vi "emballage affiche le contenu du carton_FLAT.vi"(0 "Tableau \nlots OUT":string[][](array[string]), 3 "error in":errorcluster caption="entrée d'erreur (pas d'erreur)") -> (6 "error out":errorcluster)   [LabVIEW 2020]
doc: "Affiche les pièces du même type que le produit scanné mais qui ont déjà été emballées.\nOn a la possibilité de les visualiser en sélectionnant le n° de commande et le n° du carton."
uses:
  Modules/FS/60_FS_Controles/60_FS_SetGet.ctl
panel:
  out "Nb total cartons \"théorique\"":i32
  in  "Enregistrer liste par carton (docx)":bool
  in  "Enregistrer liste par carton (txt)":bool
  out "refresh":bool
  in  "Remplacer_Valve":bool
  in  "valider":bool
  out "Total de carton dans la commande":i32
  out "Glissière 2":u8(slide)=100 caption="Identification terminé." scale=0.0..100.0
  in  "DATA cmde":T1={"n°article FAS"="12-216E-01-25 F120023 500mA 10ohm", "n° cmde FAS"="R03844/08-01.01.01", "quantité cmde"="4", "ID LIG cmde"="225540", "n° cmde client"="120565              ", "nom client"="Fluid Automat. Systems GmbH", "n° article client"="21088", "indice revision client"="      ", "société de facturation"="FAS Medic SA                            ", "langue a utiliser"="ALL"}
  out "Tab cmde GPAO":string[][](array[string])=[["12-216C-04521", "EQIFIL ", "104mA    230ohm", "03104/08-05.01.01", "3", "221769", "EMAIL VOM 01.04.08  ", "BLATTY AG", "", "      ", "Fluid Automation Systems SA             ", "ALL", "0"], ["12-216C-04521", "EQIFIL ", "104mA    230ohm", "03128/08-01.01.01", "2", "226006", "RETURN FROM VIASYS2 ", "Fluid Automat. Systems GmbH", "", "      ", "Fluid Automation Systems SA             ", "ALL", "1"], ["12-216C-04521", "EQIFIL ", "104mA    230ohm", "03130/08-01.01.01", "1", "226005", "RETURN FROM VIASYS1 ", "Fluid Automat. Systems GmbH", "", "      ", "Fluid Automation Systems SA             ", "ALL", "1"], ["12-216C-04521", "EQIFIL ", "104mA    230ohm", "03365/08-01.01.01", "4", "225536", "SANS PAPIERS GE     ", "Fluid Automat. Systems GmbH", "", "      ", "Fluid Automation Systems SA             ", "ALL", "1"], ["12-216C-04521", "EQIFIL ", "104mA    230ohm", "03570/08-02.01.01", "100", "225052", "SANS PAPIERS        ", "IMI International Sp. z o.o.", "", "      ", "Fluid Automation Systems SA             ", "ANG", "1"], ["12-216C-04521", "EQIFIL ", "104mA    230ohm", "05066/08-01.01.01", "13", "225726", "120830              ", "Fluid Automat. Systems GmbH", "", "      ", "Fluid Automation Systems SA             ", "ALL", "1"], ["12-216C-04521", "EQIFIL ", "104mA    230ohm", "05067/08-01.01.01", "11", "225727", "120831              ", "Fluid Automat. Systems GmbH", "", "      ", "Fluid Automation Systems SA             ", "ALL", "1"]]
  in  "imprimer étiquette":bool
  out "Nbr valve dans carton/commande":string
  in  "n° commande":string="6340/07-02.01.01"
  out "Pièces dans le carton":i32[](listbox)
  in  "Tableau historique":string[][](array[string])=[["MK0228606ARXA2199", "24.02.2006 11:58", "AFA", "5401/04", "1", "200"], ["MK0228606ARXA2177", "24.02.2006 12:00", "AFA", "5401/04", "1", "200"], ["MK0228606ARXA2178", "24.02.2006 12:00", "AFA", "5401/04", "1", "200"], ["MK0228606ARXA2198", "24.02.2006 12:12", "AFA", "5401/04", "1", "200"], ["MK0228606ARXA2197", "24.02.2006 12:12", "AFA", "5401/04", "1", "200"], ["MK0228606ARXA2196", "24.02.2006 12:13", "AFA", "5401/04", "1", "200"], ["MK0228606ARXA2195", "24.02.2006 12:13", "AFA", "5401/04", "1", "200"], ["MK0228606ARXA2176", "24.02.2006 12:13", "AFA", "5401/04", "1", "200"], ["MK0228606ARXA2194", "24.02.2006 12:13", "AFA", "5401/04", "1", "200"], ["MK0228606ARXA2193", "24.02.2006 12:13", "AFA", "5401/04", "1", "200"], ["MK0228606ARXA2175", "24.02.2006 12:14", "AFA", "5401/04", "1", "200"], ["MK0228606ARXA2171", "24.02.2006 12:14", "AFA", "5401/04", "1", "200"], ["MK0228606ARXA2174", "24.02.2006 12:14", "AFA", "5401/04", "1", "200"], ["MK0228606ARXA2173", "24.02.2006 12:14", "AFA", "5401/04", "1", "200"], ["MK0228606ARXA2172", "24.02.2006 12:14", "AFA", "5401/04", "1", "200"], ["MK0228606ARXA2192", "24.02.2006 12:14", "AFA", "5401/04", "1", "200"], ["MK0228606ARXA2191", "24.02.2006 12:14", "AFA", "5401/04", "1", "200"], ["MK0228606ARXA2190", "24.02.2006 12:14", "AFA", "5401/04", "1", "200"], ["MK0228606ARXA2189", "24.02.2006 12:15", "AFA", "5401/04", "1", "200"], ["MK0228606ARXA2188", "24.02.2006 12:15", "AFA", "5401/04", "1", "200"], ["MK0228606ARXB4259", "09.03.2006 17:40", "AYU", "5401/04-03.03", "5", "300"], ["MK0228606ARXB4258", "09.03.2006 17:40", "AYU", "5401/04-03.03", "5", "300"], ["MK0228606ARXB4257", "09.03.2006 17:40", "AYU", "5401/04-03.03", "5", "300"], ["MK0228606ARXB4256", "09.03.2006 17:39", "AYU", "5401/04-03.03", "5", "300"], ["MK0228606ARXB4255", "09.03.2006 17:39", "AYU", "5401/04-03.03", "5", "300"], ["MK0228606ARXB4254", "09.03.2006 17:39", "AYU", "5401/04-03.03", "5", "300"], ["MK0228606ARXB4253", "09.03.2006 17:39", "AYU", "5401/04-03.03", "5", "300"], ["MK0228606ARXB4252", "09.03.2006 17:39", "AYU", "5401/04-03.03", "5", "300"], ["MK0228606ARXB4251", "09.03.2006 17:39", "AYU", "5401/04-03.03", "5", "300"], ["MK0228606ARXB4250", "09.03.2006 17:39", "AYU", "5401/04-03.03", "5", "300"], ["MK0228606ARXB4249", "09.03.2006 17:39", "AYU", "5401/04-03.03", "5", "300"], ["MK0228606ARXB4248", "09.03.2006 17:39", "AYU", "5401/04-03.03", "5", "300"], ["MK0228606ARXB4247", "09.03.2006 17:39", "AYU", "5401/04-03.03", "5", "300"], ["MK0228606ARXB4246", "09.03.2006 17:39", "AYU", "5401/04-03.03", "5", "300"], ["MK0228606ARXB4245", "09.03.2006 17:38", "AYU", "5401/04-03.03", "5", "300"], ["MK0228606ARXB4244", "09.03.2006 17:38", "AYU", "5401/04-03.03", "5", "300"], ["MK0228606ARXB4243", "09.03.2006 17:38", "AYU", "5401/04-03.03", "5", "300"], ["MK0228606ARXB4242", "09.03.2006 17:38", "AYU", "5401/04-03.03", "5", "300"], ["MK0228606ARXB4241", "09.03.2006 17:38", "AYU", "5401/04-03.03", "5", "300"], ["MK0228606ARXB4240", "09.03.2006 17:38", "AYU", "5401/04-03.03", "5", "300"], ["MK0228606ARXB4239", "09.03.2006 17:33", "AYU", "5401/04-03.03", "4", "300"], ["MK0228606ARXB4238", "09.03.2006 17:32", "AYU", "5401/04-03.03", "4", "300"], ["MK0228606ARXB4237", "09.03.2006 17:32", "AYU", "5401/04-03.03", "4", "300"], ["MK0228606ARXB4236", "09.03.2006 17:32", "AYU", "5401/04-03.03", "4", "300"], ["MK0228606ARXB4235", "09.03.2006 17:32", "AYU", "5401/04-03.03", "4", "300"], ["MK0228606ARXB4234", "09.03.2006 17:32", "AYU", "5401/04-03.03", "4", "300"], ["MK0228606ARXB4233", "09.03.2006 17:32", "AYU", "5401/04-03.03", "4", "300"], ["MK0228606ARXB4232", "09.03.2006 17:32", "AYU", "5401/04-03.03", "4", "300"], ["MK0228606ARXB4231", "09.03.2006 17:31", "AYU", "5401/04-03.03", "4", "300"], ["MK0228606ARXB4230", "09.03.2006 17:31", "AYU", "5401/04-03.03", "4", "300"], ["MK0228606ARXB4229", "09.03.2006 17:31", "AYU", "5401/04-03.03", "4", "300"], ["MK0228606ARXB4228", "09.03.2006 17:31", "AYU", "5401/04-03.03", "4", "300"], ["MK0228606ARXB4227", "09.03.2006 17:31", "AYU", "5401/04-03.03", "4", "300"], ["MK0228606ARXB4226", "09.03.2006 17:31", "AYU", "5401/04-03.03", "4", "300"], ["MK0228606ARXB4225", "09.03.2006 17:30", "AYU", "5401/04-03.03", "4", "300"], ["MK0228606ARXB4224", "09.03.2006 17:30", "AYU", "5401/04-03.03", "4", "300"], ["MK0228606ARXB4223", "09.03.2006 17:30", "AYU", "5401/04-03.03", "4", "300"], ["MK0228606ARXB4222", "09.03.2006 17:30", "AYU", "5401/04-03.03", "4", "300"], ["MK0228606ARXB4221", "09.03.2006 17:30", "AYU", "5401/04-03.03", "4", "300"], ["MK0228606ARXB4220", "09.03.2006 17:30", "AYU", "5401/04-03.03", "4", "300"], ["MK0228606ARXB4219", "09.03.2006 17:24", "AYU", "5401/04-03.03", "3", "300"], ["MK0228606ARXB4218", "09.03.2006 17:23", "AYU", "5401/04-03.03", "3", "300"], ["MK0228606ARXB4217", "09.03.2006 17:23", "AYU", "5401/04-03.03", "3", "300"], ["MK0228606ARXB4216", "09.03.2006 17:23", "AYU", "5401/04-03.03", "3", "300"], ["MK0228606ARXB4215", "09.03.2006 17:23", "AYU", "5401/04-03.03", "3", "300"], ["MK0228606ARXB4214", "09.03.2006 17:23", "AYU", "5401/04-03.03", "3", "300"], ["MK0228606ARXB4213", "09.03.2006 17:23", "AYU", "5401/04-03.03", "3", "300"], ["MK0228606ARXB4212", "09.03.2006 17:22", "AYU", "5401/04-03.03", "3", "300"], ["MK0228606ARXB4211", "09.03.2006 17:21", "AYU", "5401/04-03.03", "3", "300"], ["MK0228606ARXB4210", "09.03.2006 17:21", "AYU", "5401/04-03.03", "3", "300"], ["MK0228606ARXB4209", "09.03.2006 17:21", "AYU", "5401/04-03.03", "3", "300"], ["MK0228606ARXB4208", "09.03.2006 17:20", "AYU", "5401/04-03.03", "3", "300"], ["MK0228606ARXB4207", "09.03.2006 17:20", "AYU", "5401/04-03.03", "3", "300"], ["MK0228606ARXB4206", "09.03.2006 17:20", "AYU", "5401/04-03.03", "3", "300"], ["MK0228606ARXB4205", "09.03.2006 17:20", "AYU", "5401/04-03.03", "3", "300"], ["MK0228606ARXB4204", "09.03.2006 17:20", "AYU", "5401/04-03.03", "3", "300"], ["MK0228606ARXB4203", "09.03.2006 17:20", "AYU", "5401/04-03.03", "3", "300"], ["MK0228606ARXB4202", "09.03.2006 17:19", "AYU", "5401/04-03.03", "3", "300"], ["MK0228606ARXB4201", "09.03.2006 17:19", "AYU", "5401/04-03.03", "3", "300"], ["MK0228606ARXB4200", "09.03.2006 17:18", "AYU", "5401/04-03.03", "3", "300"], ["MK0228606ARXB4199", "09.03.2006 17:12", "AYU", "5401/04-03.03", "2", "300"], ["MK0228606ARXB4198", "09.03.2006 17:11", "AYU", "5401/04-03.03", "2", "300"], ["MK0228606ARXB4197", "09.03.2006 17:11", "AYU", "5401/04-03.03", "2", "300"], ["MK0228606ARXB4196", "09.03.2006 17:11", "AYU", "5401/04-03.03", "2", "300"], ["MK0228606ARXB4195", "09.03.2006 17:11", "AYU", "5401/04-03.03", "2", "300"], ["MK0228606ARXB4194", "09.03.2006 17:11", "AYU", "5401/04-03.03", "2", "300"], ["MK0228606ARXB4193", "09.03.2006 17:11", "AYU", "5401/04-03.03", "2", "300"], ["MK0228606ARXB4192", "09.03.2006 17:10", "AYU", "5401/04-03.03", "2", "300"], ["MK0228606ARXB4191", "09.03.2006 17:10", "AYU", "5401/04-03.03", "2", "300"], ["MK0228606ARXB4190", "09.03.2006 17:10", "AYU", "5401/04-03.03", "2", "300"], ["MK0228606ARXB4189", "09.03.2006 17:10", "AYU", "5401/04-03.03", "2", "300"], ["MK0228606ARXB4188", "09.03.2006 17:10", "AYU", "5401/04-03.03", "2", "300"], ["MK0228606ARXB4187", "09.03.2006 17:10", "AYU", "5401/04-03.03", "2", "300"], ["MK0228606ARXB4186", "09.03.2006 17:10", "AYU", "5401/04-03.03", "2", "300"], ["MK0228606ARXB4185", "09.03.2006 17:10", "AYU", "5401/04-03.03", "2", "300"], ["MK0228606ARXB4184", "09.03.2006 17:09", "AYU", "5401/04-03.03", "2", "300"], ["MK0228606ARXB4183", "09.03.2006 17:09", "AYU", "5401/04-03.03", "2", "300"], ["MK0228606ARXB4182", "09.03.2006 17:09", "AYU", "5401/04-03.03", "2", "300"], ["MK0228606ARXB4181", "09.03.2006 17:08", "AYU", "5401/04-03.03", "2", "300"], ["MK0228606ARXB4180", "09.03.2006 17:08", "AYU", "5401/04-03.03", "2", "300"], ["MK0228606ARXB4179", "09.03.2006 17:01", "AYU", "5401/04-03.03", "1", "300"], ["MK0228606ARXB4178", "09.03.2006 17:01", "AYU", "5401/04-03.03", "1", "300"], ["MK0228606ARXB4177", "09.03.2006 17:01", "AYU", "5401/04-03.03", "1", "300"], ["MK0228606ARXB4176", "09.03.2006 17:01", "AYU", "5401/04-03.03", "1", "300"], ["MK0228606ARXB4175", "09.03.2006 17:00", "AYU", "5401/04-03.03", "1", "300"], ["MK0228606ARXB4174", "09.03.2006 17:00", "AYU", "5401/04-03.03", "1", "300"], ["MK0228606ARXB4173", "09.03.2006 17:00", "AYU", "5401/04-03.03", "1", "300"], ["MK0228606ARXB4172", "09.03.2006 17:00", "AYU", "5401/04-03.03", "1", "300"], ["MK0228606ARXB4171", "09.03.2006 17:00", "AYU", "5401/04-03.03", "1", "300"], ["MK0228606ARXB4170", "09.03.2006 16:57", "AYU", "5401/04-03.03", "1", "300"], ["MK0228606ARXB4169", "09.03.2006 16:57", "AYU", "5401/04-03.03", "1", "300"], ["MK0228606ARXB4168", "09.03.2006 16:56", "AYU", "5401/04-03.03", "1", "300"], ["MK0228606ARXB4167", "09.03.2006 16:56", "AYU", "5401/04-03.03", "1", "300"], ["MK0228606ARXB4166", "09.03.2006 16:56", "AYU", "5401/04-03.03", "1", "300"], ["MK0228606ARXB4165", "09.03.2006 16:55", "AYU", "5401/04-03.03", "1", "300"], ["MK0228606ARXB4164", "09.03.2006 16:55", "AYU", "5401/04-03.03", "1", "300"], ["MK0228606ARXB4163", "09.03.2006 16:55", "AYU", "5401/04-03.03", "1", "300"], ["MK0228606ARXB4162", "09.03.2006 16:54", "AYU", "5401/04-03.03", "1", "300"], ["MK0228606ARXB4161", "09.03.2006 16:54", "AYU", "5401/04-03.03", "1", "300"], ["MK0228606ARXB4160", "09.03.2006 16:52", "AYU", "5401/04-03.03", "1", "300"], ["MK0228606ARXB4158", "10.03.2006 08:35", "AYU", "5401/04-03.03", "1", "300"], ["MK0228606ARXB4159", "10.03.2006 08:34", "AYU", "5401/04-03.03", "1", "300"]]
  in  "quitter":bool
  in  "N° du carton":i16=1 min=0 max=2
  # "Saisir le n° de la commande"
  # "Seul un responsable peut ré-imprimer\nune étiquette d'emballage"
  # "Enregistrer liste par carton"
  # "Option vérouillé par un mot de passe"
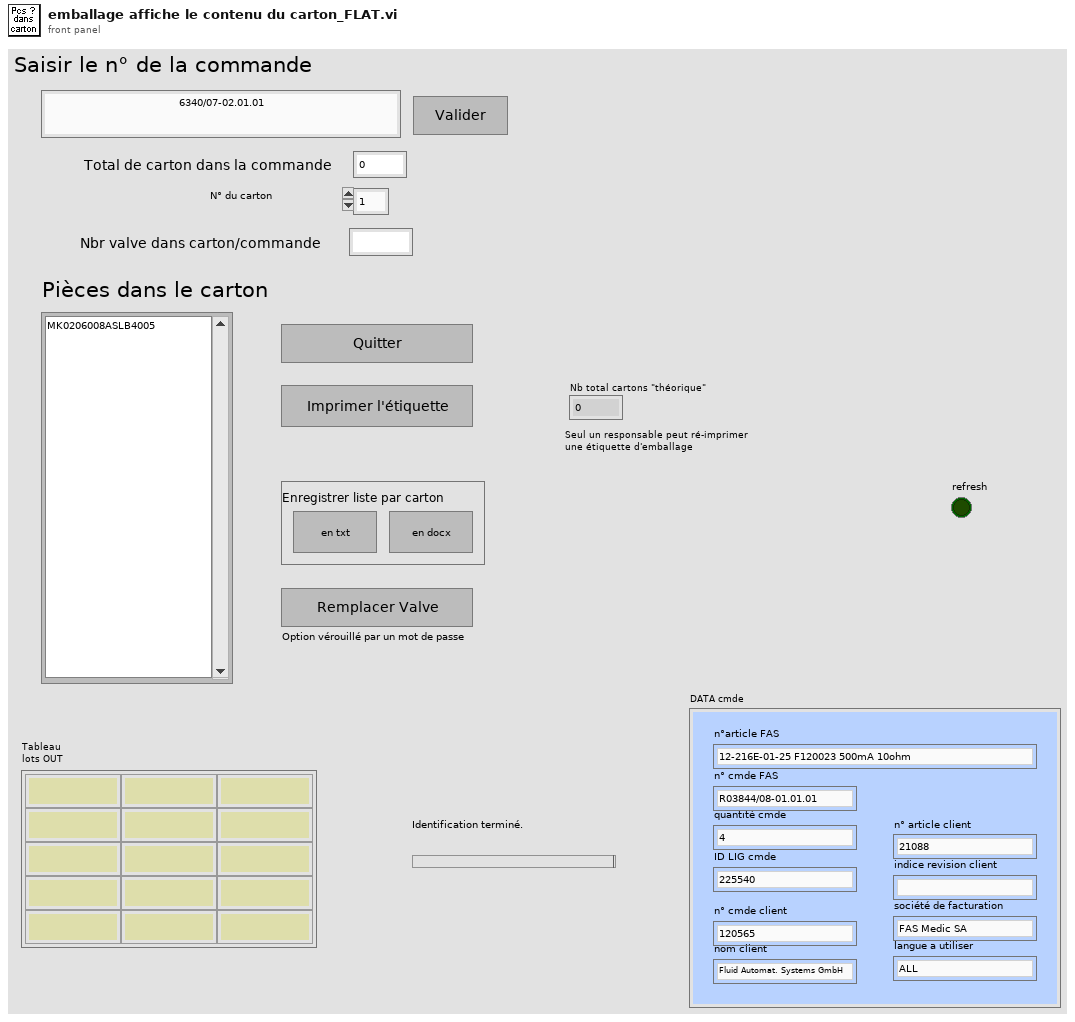
[diagram p1: front panel]
types:
  T1 = typedef "DATA commande.ctl" = cluster{"n°article FAS":string, "n° cmde FAS":string, "quantité cmde":string, "ID LIG cmde":string, "n° cmde client":string, "nom client":string, "n° article client":string, "indice revision client":string, "société de facturation":string, "langue a utiliser":string}
  T2 = typedef "60_FS_SetGet.ctl" = enum16{"set", "get"}
  T3 = enum8{"Enabled", "Disabled", "Disabled and Grayed Out"}
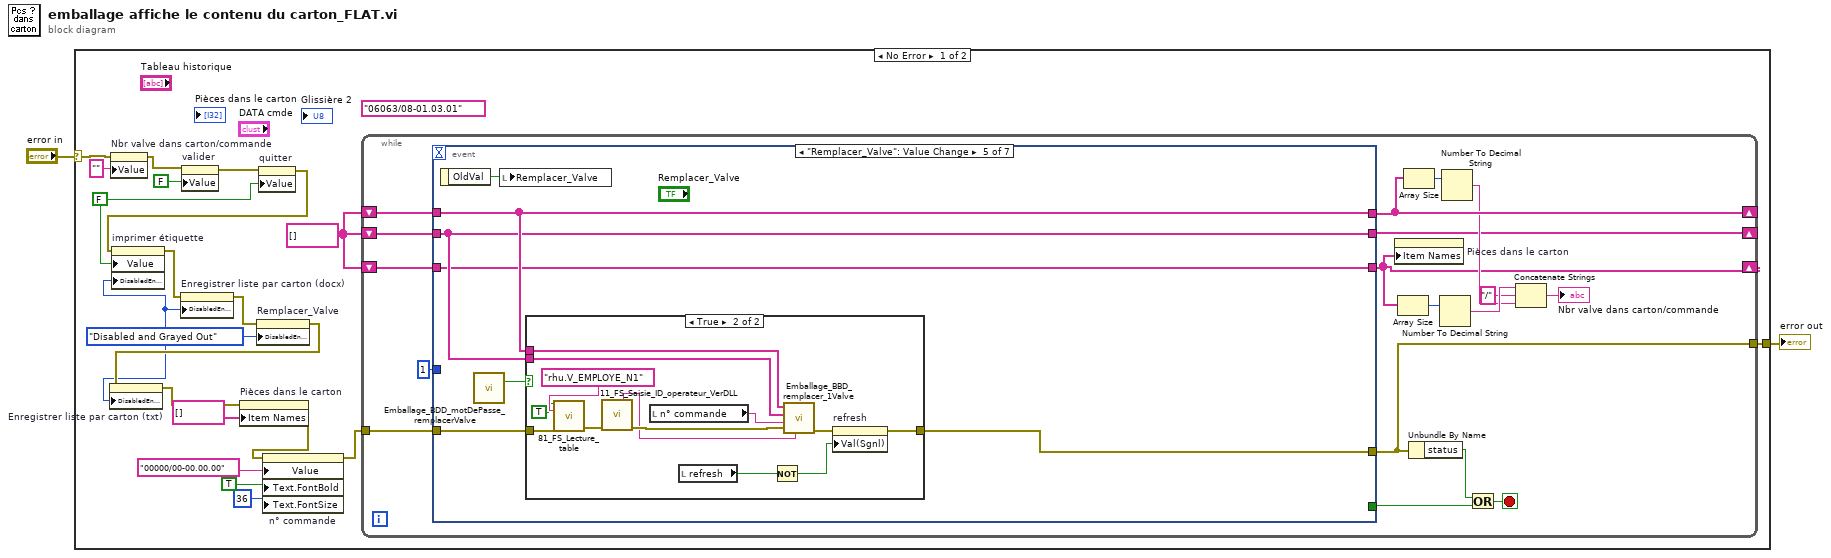
[diagram p0: block diagram]
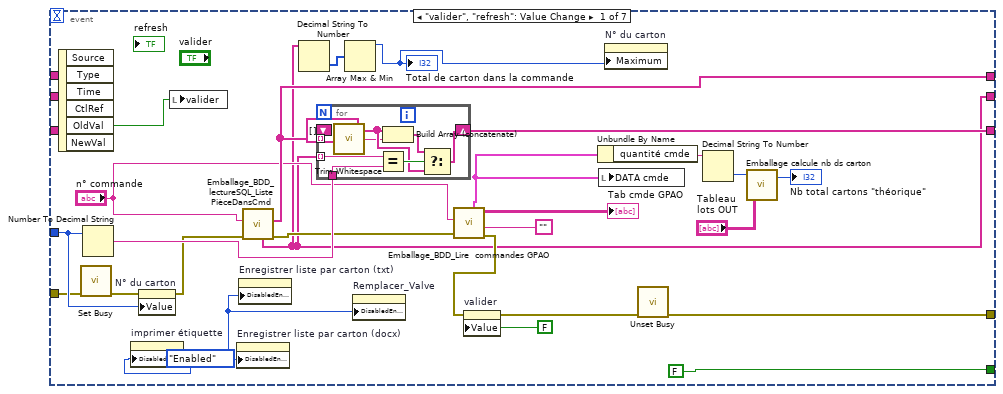
[diagram p2: hidden frame]
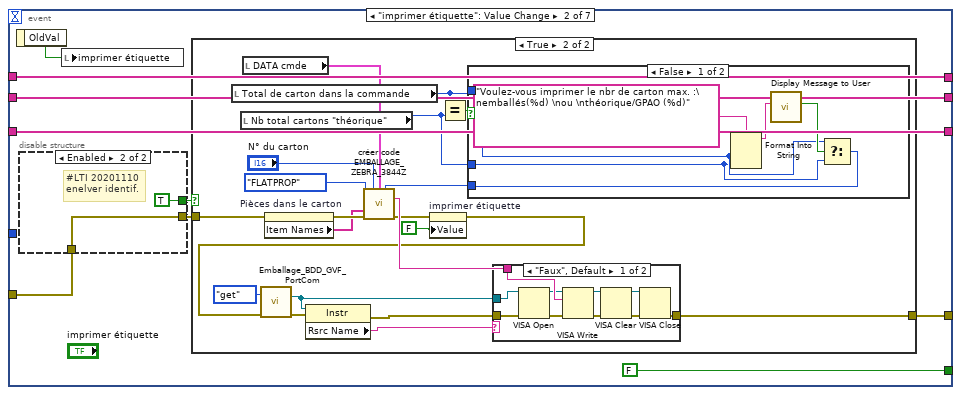
[diagram p3: hidden frame]
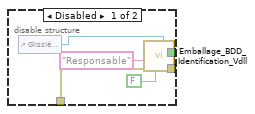
[diagram p4: hidden frame]
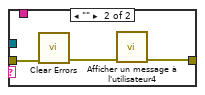
[diagram p7: hidden frame]
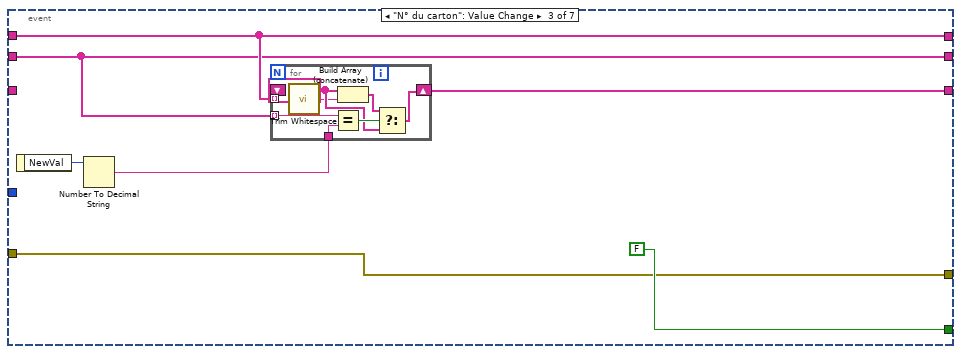
[diagram p8: hidden frame]
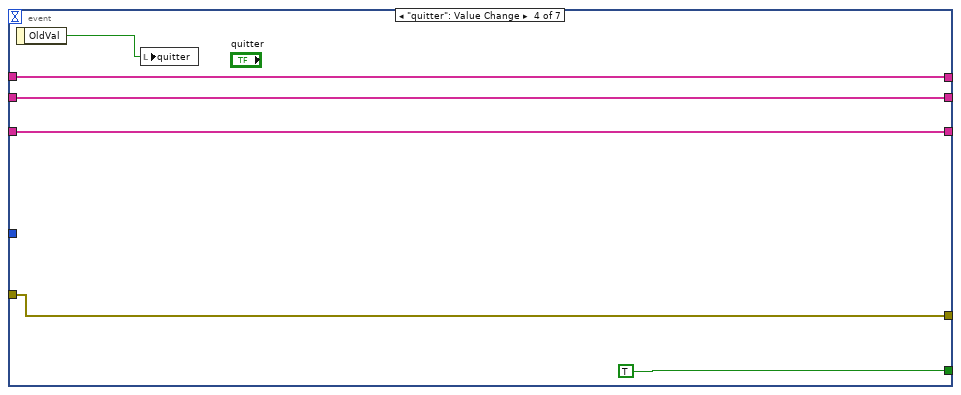
[diagram p9: hidden frame]
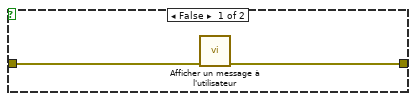
[diagram p10: hidden frame]
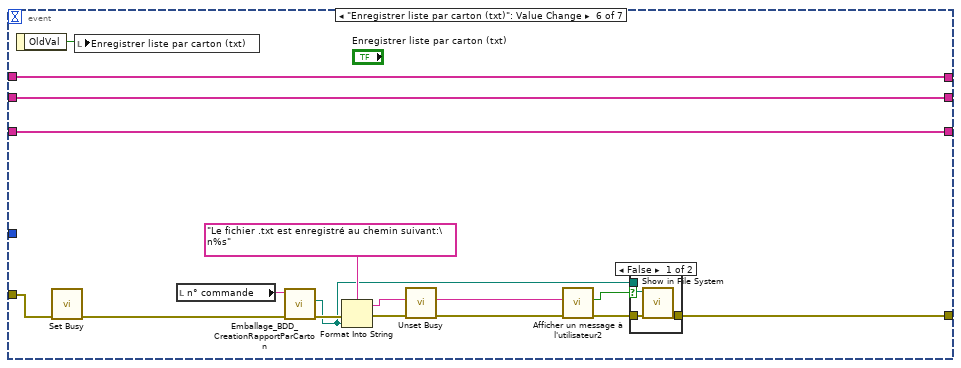
[diagram p11: hidden frame]
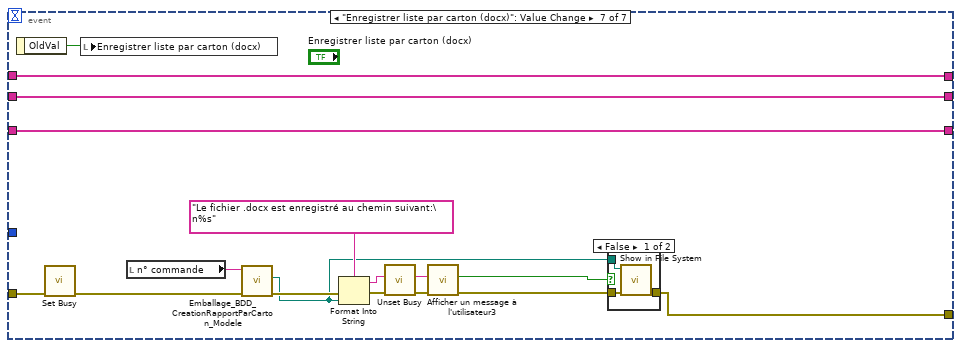
[diagram p13: hidden frame]
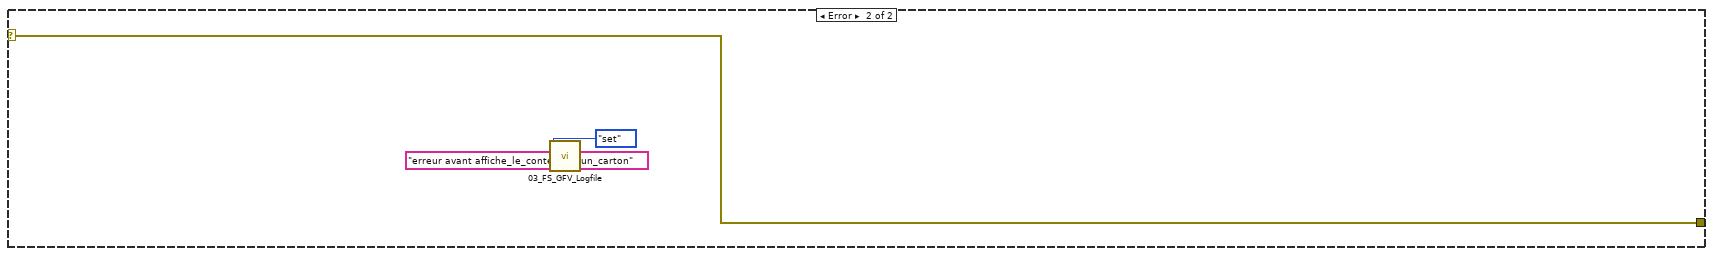
[diagram p15: hidden frame]
diagram:
  n1 = case shown="No Error" "error in" {
    selector: "error in" -> [w11 w220]
    tunnel: [w22 w220] -> w1
    frame No Error {
      w4 = T3."Disabled and Grayed Out" ("Désactivé")
      w15 = string[] [] ("Liste n° pièces de la cmde")
      (unwired) "06063/08-01.03.01" ("N° Commande")
      w17 = FALSE
      n2 = property on="Nbr valve dans carton/commande" class="Str"(error in=w11, "Value"="" ("Nbr valve dans carton/commande")) -> (error out=w8:errorcluster)  [unwired: 1 in, 1 out]
      n3 = property on="valider" class="Bool (strict)"(error in=w8, "Value"=FALSE ("valider")) -> (error out=w10:errorcluster)  [unwired: 1 in, 1 out]
      n4 = property on="quitter" class="Bool (strict)"(error in=w10, "Value"=w17) -> (error out=w16:errorcluster)  [unwired: 1 in, 1 out]
      n5 = property on="imprimer étiquette" class="Bool (strict)"(error in=w16, "Value"=w17, "DisabledEnum"=w4) -> (error out=w6:errorcluster)  [unwired: 1 in, 1 out]
      n6 = property on="Enregistrer liste par carton (docx)" class="Bool (strict)"(error in=w6, "DisabledEnum"=w4) -> (error out=w5:errorcluster)  [unwired: 1 in, 1 out]
      n7 = property on="Remplacer_Valve" class="Bool (strict)"(error in=w5, "DisabledEnum"=w4) -> (error out=w7:errorcluster)  [unwired: 1 in, 1 out]
      n8 = property on="Enregistrer liste par carton (txt)" class="Bool (strict)"(error in=w7, "DisabledEnum"=w4) -> (error out=w3:errorcluster)  [unwired: 1 in, 1 out]
      n9 = property on="Pièces dans le carton" class="LstBox (strict)"(error in=w3, "Item Names"=string[] [] ("Noms d'éléments")) -> (error out=w13:errorcluster)  [unwired: 1 in, 1 out]
      n10 = property on="n° commande" class="Str"(error in=w13, "Value"="00000/00-00.00.00" ("n° commande"), "Text.FontBold"=TRUE ("Texte.Police : gras"), "Text.FontSize"=u32 36 ("Texte.Police : taille")) -> (error out=w18:errorcluster)  [unwired: 1 in, 1 out]
      n11 = while {
        tunnel: w18 -> [w37]
        tunnel: [w36] -> w22
        shift-right: [w32] -> _
        shift-left: w15 -> [w35]
        shift-right: [w23] -> _
        shift-left: w15 -> [w34]
        shift-right: [w25] -> _
        shift-left: w15 -> [w24]
        stop <- w40 stop-if-true
        n12 = event shown="[4] \"Remplacer_Valve\": Value Change" {
          selector: _ -> [_ _ _ _ _ _ _]
          dyn-events: _ -> [_ _ _ _ _ _ _]
          timeout: _ -> [_ _ _ _ _ _ _]
          tunnel: [FALSE FALSE FALSE TRUE _ _ _] -> w39
          tunnel: i16 1 ("N° du carton") -> [w61 _ _ _ _ _ _]
          tunnel: w37 -> [w51 w80 w136 w152 w162 w188 w208]
          tunnel: [w49 w83 w136 w152 w161 w180 w200] -> w36
          tunnel: [w66 w79 w135 w154 w159 w186 w206] -> w32
          tunnel: [w55 w76 w134 w153 w158 w185 w205] -> w23
          tunnel: w35 -> [_ w79 w135 w154 w159 w186 w206]
          tunnel: w34 -> [_ w76 w134 w153 w158 w185 w205]
          tunnel: [w63 w78 w137 w151 w157 w184 w204] -> w25
          tunnel: w24 -> [_ w78 _ w151 w157 w184 w204]
          event "valider", "refresh": Value Change {
            w47 = T3."Enabled" ("Désactivé")
            n13 = event-data() -> ("OldVal"=w52:bool)  [unwired: 1 in, 5 out]
            n14 = call <vilib>:"Set Busy.vi"("error in (no error)"=w51) -> ("error out"=w50:errorcluster)  [unwired: 9 in, 1 out]
            n15 = Number To Decimal String(number=w61) -> (decimal integer string=w65:string)  [unwired: 1 in]
            n16 = property on="imprimer étiquette" class="Bool (strict)"("DisabledEnum"=w47) -> ()  [unwired: 2 in, 2 out]
            n17 = property on="N° du carton" class="DigNum (strict)"(error in=w50, "Value"=w61) -> (error out=w62:errorcluster)  [unwired: 1 in, 1 out]
            n18 = local write "valider"(w52) -> ()
            n19 = property on="Enregistrer liste par carton (docx)" class="Bool (strict)"("DisabledEnum"=w47) -> ()  [unwired: 2 in, 2 out]
            n20 = property on="Enregistrer liste par carton (txt)" class="Bool (strict)"("DisabledEnum"=w47) -> ()  [unwired: 2 in, 2 out]
            n21 = call "Emballage_BDD_lectureSQL_Liste PièceDansCmd.vi"("Error in"=w62, "NO_CDEVAL"="n° commande") -> ("Error out"=w58:errorcluster, "Liste n° pièces de la cmde"=w66:string[], "Carton"=w55:string[])  [unwired: 5 in, 2 out]
            n22 = Decimal String To Number(string=w55) -> (number=w54:i32[])  [unwired: 2 in, 1 out]
            n23 = for {
              tunnel: w66 -> [w69] mode=indexing
              tunnel: w55 -> [w75] mode=indexing
              tunnel: w65 -> [w74]
              shift-right: [w72] -> w63
              shift-left: string[] [] -> [w70]
              n24 = call <vilib>:"Trim Whitespace.vi"("string"=w69) -> ("trimmed string"=w68:string)  [unwired: 1 in]
              n25 = Equal?(x=w75, y=w74) -> (x = y?=w73:bool)
              n26 = Build Array (concatenate)(w70, w68) -> (w71:string[])
              n27 = Select(t=w71, s=w73, f=w70) -> (s? t:f=w72:string[])
            }
            n28 = Array Max & Min(array=w54) -> (max value=w53:i32)  [unwired: 3 out]
            "Total de carton dans la commande" <- w53
            n29 = property on="Remplacer_Valve" class="Bool (strict)"("DisabledEnum"=w47) -> ()  [unwired: 2 in, 2 out]
            n30 = call "Emballage_BDD_Lire  commandes GPAO.vi"("error in"=w58, "article"="", "Numéro commande"="n° commande") -> ("error out"=w57:errorcluster, "Tab cmde GPAO"=→"Tab cmde GPAO":string[][], "DATA cmde"=w44:T1)  [unwired: 3 in, 3 out]
            n31 = property on="valider" class="Bool (strict)"(error in=w57, "Value"=FALSE ("valider")) -> (error out=w48:errorcluster)  [unwired: 1 in, 1 out]
            n32 = Unbundle By Name(w44) -> ("quantité cmde"=w46:string)
            n33 = local write "DATA cmde"(w44) -> ()
            n34 = property on="N° du carton" class="DigNum (strict)"("Maximum"=w53) -> ()  [unwired: 2 in, 2 out]
            n35 = call <vilib>:"Unset Busy.vi"("error in (no error)"=w48) -> ("error out"=w49:errorcluster)  [unwired: 10 in]
            n36 = Decimal String To Number(string=w46) -> (number=w43:i32)  [unwired: 2 in, 1 out]
            n37 = call "Emballage calcule nb ds carton.vi"("Tableau \nlots OUT"="Tableau \nlots OUT", "Quantité de la cmde"=w43) -> ("Nb total cartons"=→"Nb total cartons \"théorique\"":i32)  [unwired: 1 in, 1 out]
          }
          event "imprimer étiquette": Value Change {
            n38 = event-data() -> ("OldVal"=w77:bool)  [unwired: 1 in]
            n39 = disable-structure shown="Enabled" {
              disable-tunnel: [w87 w92] -> w82
              disable-tunnel: [w86 TRUE ("OK")] -> w81
              disable-tunnel: w80 -> [w85 w92]
              frame Disabled {
                n40 = control-ref of="Glissière 2"() -> (w88:refnum<vi>)
                n41 = call "Emballage_BDD_Identification_Vdll.vi"("Glissière"=w88, "lecture seul possible ?"=FALSE, "error in"=w85, "Posage choisi"="Responsable") -> ("error Out"=w87:errorcluster, "OK"=w86:bool)  [unwired: 3 in, 3 out]
              }
              frame Enabled {
                # "#LTI 20201110\nenelver identif."
              }
            }
            n42 = local write "imprimer étiquette"(w77) -> ()
            n43 = case shown="True" w81 {
              tunnel: [w93 w113] -> w83
              tunnel: w82 -> [w93 w108]
              frame False {
              }
              frame True {
                n44 = local read "Total de carton dans la commande"() -> (w95:i32)
                n45 = local read "Nb total cartons \"théorique\""() -> (w94:i32)
                n46 = local read "DATA cmde"() -> (w109:T1)
                n47 = property on="Pièces dans le carton" class="LstBox (strict)"(error in=w108) -> (error out=w107:errorcluster, "Item Names"=w104:string[])  [unwired: 1 in, 1 out]
                n48 = Equal?(x=w95, y=w94) -> (x = y?=w97:bool)
                n49 = case shown="False" w97 {
                  tunnel: [w114 w120] -> w96
                  tunnel: w95 -> [w116 w120]
                  tunnel: w94 -> [w115 _]
                  frame False {
                    n50 = Format Into String(format string="Voulez-vous imprimer le nbr de carton max. :\nemballés(%d) \nou \nthéorique/GPAO (%d)" ("Message"), w116, w115) -> (resulting string=w119:string)  [unwired: 2 in, 1 out]
                    n51 = call "Display Message to User"("Message"=w119) -> ("Emballés"=w117:bool)  [unwired: 9 in, 1 out]
                    n52 = Select(t=w116, s=w117, f=w115) -> (s? t:f=w114:i32)
                  }
                  frame True {
                  }
                }
                n53 = call "créer code EMBALLAGE_ZEBRA_3844Z.vi"("DIVISION"=enum16{"FLATPROP", "MEDIC"}."FLATPROP", "N° carton"="N° du carton", "DATA cmde"=w109, "Nb total cartons"=w96, "Tableau n° valves"=w104, "error in (no error)"=w107) -> ("chaine  à écrire"=w112:string, "error out"=w106:errorcluster)  [unwired: 6 in, 2 out]
                n54 = property on="imprimer étiquette" class="Bool (strict)"(error in=w106, "Value"=FALSE ("imprimmer étiquette")) -> (error out=w103:errorcluster)  [unwired: 1 in, 1 out]
                n55 = call "Emballage_BDD_GVF_PortCom.vi"("Énum"=enum16{"get", "set"}."get", "Error in"=w103) -> ("PortCom imprimante OUT"=w100:refnum<visa-resource-name>, "Error out"=w101:errorcluster)  [unwired: 7 in, 5 out]
                n56 = property class="Instr"(reference=w100, error in=w101) -> (error out=w99:errorcluster, "Rsrc Name"=w98:string)  [unwired: 1 out]
                n57 = case shown="\"Faux\", Default" w98 {
                  tunnel: [w130 w131] -> w113
                  tunnel: w112 -> [w125 _]
                  tunnel: w99 -> [w124 w133]
                  tunnel: w100 -> [w121 _]
                  frame "Faux", Default {
                    n58 = VISA Open(error in (no error)=w124, VISA resource name=w121) -> (VISA resource name=w122:refnum<visa-resource-name>, error out=w123:errorcluster)  [unwired: 3 in]
                    n59 = VISA Write(VISA resource name=w122, write buffer=w125, error in (no error)=w123) -> (VISA resource name out=w126:refnum<visa-resource-name>, error out=w127:errorcluster)  [unwired: 1 out]
                    n60 = VISA Clear(VISA resource name=w126, error in (no error)=w127) -> (VISA resource name out=w128:refnum<visa-resource-name>, error out=w129:errorcluster)
                    n61 = VISA Close(VISA resource name=w128, error in (no error)=w129) -> (error out=w130:errorcluster)
                  }
                  frame "" {
                    n62 = call <vilib>:"Clear Errors.vi"("error in (no error)"=w133) -> ("error out"=w132:errorcluster)  [unwired: 5 in, 1 out]
                    n63 = call "Afficher un message à l'utilisateur4"("error in (no error)"=w132) -> ("error out"=w131:errorcluster)  [unwired: 9 in, 1 out]
                  }
                }
              }
            }
          }
          event "N° du carton": Value Change {
            n64 = event-data() -> ("NewVal"=w140:i16)  [unwired: 1 in]
            n65 = Number To Decimal String(number=w140) -> (decimal integer string=w139:string)  [unwired: 1 in]
            n66 = for {
              tunnel: w135 -> [w143] mode=indexing
              tunnel: w134 -> [w149] mode=indexing
              tunnel: w139 -> [w148]
              shift-right: [w146] -> w137
              shift-left: string[] [] -> [w144]
              n67 = call <vilib>:"Trim Whitespace.vi"("string"=w143) -> ("trimmed string"=w142:string)  [unwired: 1 in]
              n68 = Equal?(x=w149, y=w148) -> (x = y?=w147:bool)
              n69 = Build Array (concatenate)(w144, w142) -> (w145:string[])
              n70 = Select(t=w145, s=w147, f=w144) -> (s? t:f=w146:string[])
            }
          }
          event "quitter": Value Change {
            n71 = event-data() -> ("OldVal"=w150:bool)  [unwired: 1 in]
            n72 = local write "quitter"(w150) -> ()
          }
          event "Remplacer_Valve": Value Change {
            n73 = event-data() -> ("OldVal"=w156:bool)  [unwired: 1 in]
            n74 = call "Emballage_BDD_motDePasse_remplacerValve.vi"() -> ("Booléen"=w160:bool)  [unwired: 11 in]
            n75 = local write "Remplacer_Valve"(w156) -> ()
            n76 = case shown="True" w160 {
              tunnel: w159 -> [_ w177]
              tunnel: w158 -> [_ w176]
              tunnel: w162 -> [w164 w166]
              tunnel: [w163 w173] -> w161
              frame False {
                n77 = call "Afficher un message à l'utilisateur"("error in (no error)"=w164) -> ("error out"=w163:errorcluster)  [unwired: 9 in, 1 out]
              }
              frame True {
                n78 = call "81_FS_Lecture_table.vi"("T:VSX/F:PLZ"=TRUE, "table à charger"="rhu.V_EMPLOYE_N1", "error in (no error)"=w166) -> ("error out"=w167:errorcluster)  [unwired: 8 in, 4 out]
                n79 = call "11_FS_Saisie_ID_operateur_VerDLL.vi"("error in (no error)"=w167) -> ("ID_EMPLOYE"=w165:string, "error out"=w168:errorcluster)  [unwired: 9 in, 4 out]
                n80 = local read "n° commande"() -> (w175:string)
                n81 = local read "refresh"() -> (w172:bool)
                n82 = Not(x=w172) -> (.not. x?=w171:bool)
                n83 = call "Emballage_BBD_remplacer_1Valve.vi"("ID_UTILISATEUR_GPAO"=w165, "Error in"=w168, "No Commande :"=w175, "Liste Carton"=w176, "Liste n° pièces de la cmde"=w177) -> ("Error out"=w174:errorcluster)  [unwired: 6 in]
                n84 = property on="refresh" class="Bool (strict)"(error in=w174, "Val(Sgnl)"=w171) -> (error out=w173:errorcluster)  [unwired: 1 in, 1 out]
              }
            }
          }
          event "Enregistrer liste par carton (txt)": Value Change {
            n85 = event-data() -> ("OldVal"=w190:bool)  [unwired: 1 in]
            n86 = call <vilib>:"Set Busy.vi"("error in (no error)"=w188) -> ("error out"=w187:errorcluster)  [unwired: 9 in, 1 out]
            n87 = local write "Enregistrer liste par carton (txt)"(w190) -> ()
            n88 = local read "n° commande"() -> (w193:string)
            n89 = call "Emballage_BDD_CreationRapportParCarton.vi"("error in (no error)"=w187, "N° Cmd"=w193) -> ("error out"=w189:errorcluster, "chemin complet"=w179:path)  [unwired: 6 in, 2 out]
            n90 = Format Into String(format string="Le fichier .txt est enregistré au chemin suivant:\n%s" ("Message"), error in=w189, w179) -> (resulting string=w191:string, error out=w183:errorcluster)  [unwired: 1 in]
            n91 = call <vilib>:"Unset Busy.vi"("error in (no error)"=w183) -> ("error out"=w182:errorcluster)  [unwired: 10 in]
            n92 = call "Afficher un message à l'utilisateur2"("error in (no error)"=w182, "Message"=w191) -> ("error out"=w181:errorcluster, "OK"=w178:bool)  [unwired: 8 in]
            n93 = case shown="False" w178 {
              tunnel: w181 -> [w196 w197]
              tunnel: [w195 w197] -> w180
              tunnel: w179 -> [w194 _]
              frame False {
                n94 = call <vilib>:"Show in File System.vi"("error in (no error)"=w196, "file or directory path"=w194) -> ("error out"=w195:errorcluster)  [unwired: 9 in]
              }
              frame True {
              }
            }
          }
          event "Enregistrer liste par carton (docx)": Value Change {
            n95 = event-data() -> ("OldVal"=w213:bool)  [unwired: 1 in]
            n96 = call <vilib>:"Set Busy.vi"("error in (no error)"=w208) -> ("error out"=w207:errorcluster)  [unwired: 9 in, 1 out]
            n97 = local write "Enregistrer liste par carton (docx)"(w213) -> ()
            n98 = local read "n° commande"() -> (w210:string)
            n99 = call "Emballage_BDD_CreationRapportParCarton_Modele.vi"("error in (no error)"=w207, "N° Cmd"=w210) -> ("error out"=w209:errorcluster, "chemin complet"=w198:path)  [unwired: 8 in]
            n100 = Format Into String(format string="Le fichier .docx est enregistré au chemin suivant:\n%s" ("Message"), error in=w209, w198) -> (resulting string=w212:string, error out=w203:errorcluster)  [unwired: 1 in]
            n101 = call <vilib>:"Unset Busy.vi"("error in (no error)"=w203) -> ("error out"=w202:errorcluster)  [unwired: 10 in]
            n102 = call "Afficher un message à l'utilisateur3"("error in (no error)"=w202, "Message"=w212) -> ("error out"=w201:errorcluster, "OK"=w199:bool)  [unwired: 8 in]
            n103 = case shown="False" w199 {
              tunnel: w201 -> [w216 w217]
              tunnel: [w215 w217] -> w200
              tunnel: w198 -> [w214 _]
              frame False {
                n104 = call <vilib>:"Show in File System.vi"("error in (no error)"=w216, "file or directory path"=w214) -> ("error out"=w215:errorcluster)  [unwired: 9 in]
              }
              frame True {
              }
            }
          }
        }
        n105 = property on="Pièces dans le carton" class="LstBox (strict)"("Item Names"=w25) -> ()  [unwired: 2 in, 2 out]
        n106 = Array Size(array=w25) -> (size(s)=w30:i32)
        n107 = Array Size(array=w32) -> (size(s)=w31:i32)
        n108 = Unbundle By Name(w36) -> ("status"=w38:bool)
        n109 = Number To Decimal String(number=w30) -> (decimal integer string=w29:string)  [unwired: 1 in]
        n110 = Number To Decimal String(number=w31) -> (decimal integer string=w27:string)  [unwired: 1 in]
        n111 = Or(x=w38, y=w39) -> (x .or. y?=w40:bool)
        n112 = Concatenate Strings(w29, "/" ("chaîne"), w27) -> (→"Nbr valve dans carton/commande":string)
      }
    }
    frame Error {
      n113 = call "03_FS_GFV_Logfile.vi"("Chaîne"="erreur avant affiche_le_contenu_d_un_carton", "States"=60_FS_SetGet."set") -> ()  [unwired: 8 in, 2 out]
    }
  }
  "error out" <- w1
